vi "Insert Specifical Controls to [8,8] Array.vi"(7 "controls references":refnum<vi>[](array[refnum]), 8 "error in":errorcluster {"code" format="%.0x"}, 9 "2-D controls references":refnum<vi>[][](array[refnum]), 10 "indicators":refnum<vi>[](array[refnum]), 11 "controls":refnum<vi>[](array[refnum])) -> (0 "error out":errorcluster {"code" format="%.0x"}, 1 "2-D controls references out":refnum<vi>[][](array[refnum]), 2 "indicators out":refnum<vi>[](array[refnum]), 3 "controls out":refnum<vi>[](array[refnum]), 4 "controls references out":refnum<vi>[](array[refnum]))   [LabVIEW 2018, in "NISAST VI Scripting.lvlib" / "VI.lvlib" / "Front Panel.lvlib"]
uses:
  Front Panel.lvlib
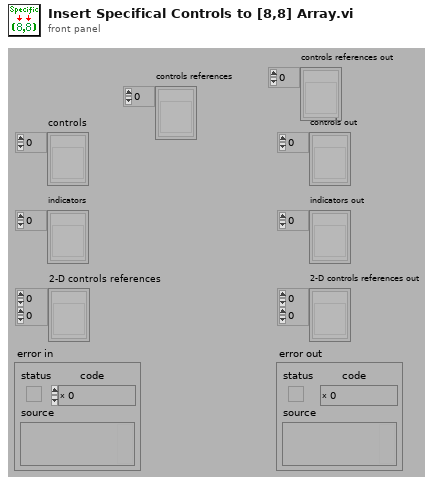
[diagram p1: front panel]
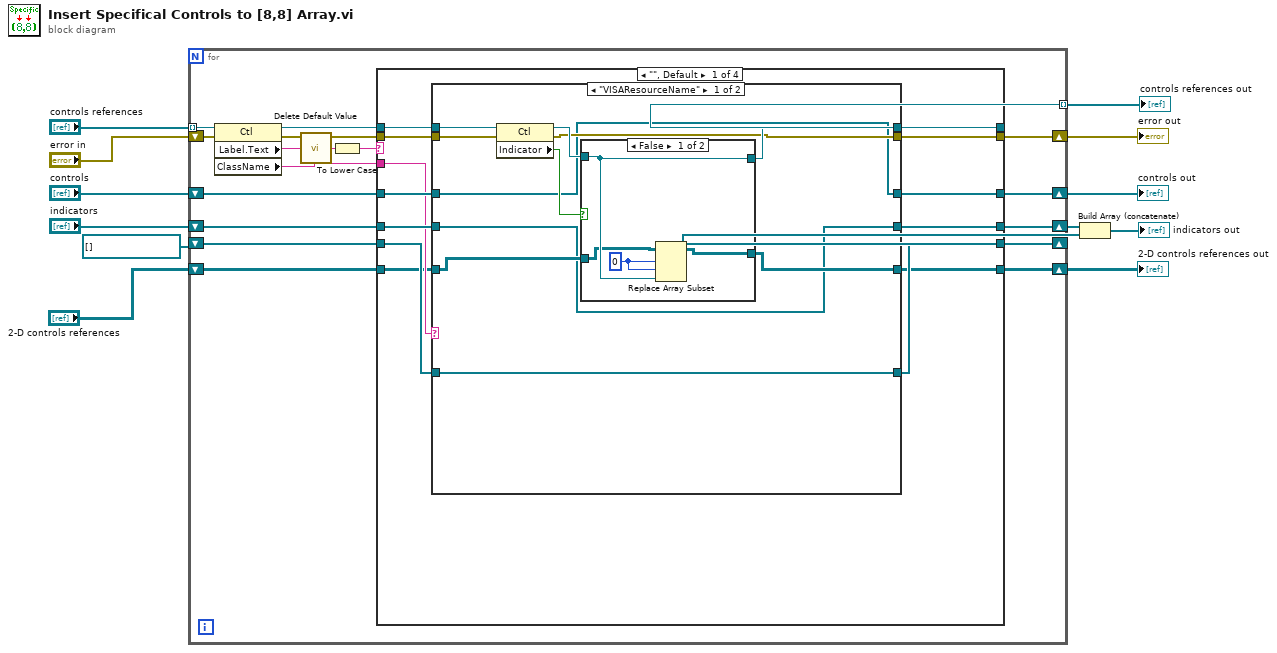
[diagram p0: block diagram]
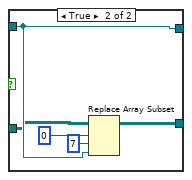
[diagram p2: hidden frame]
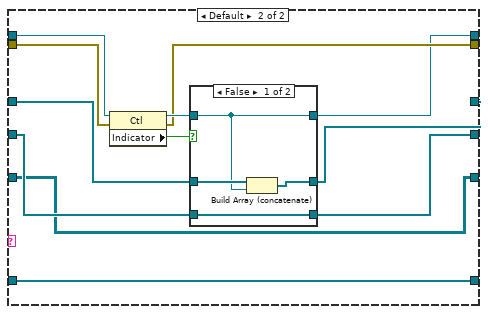
[diagram p3: hidden frame]
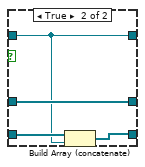
[diagram p4: hidden frame]
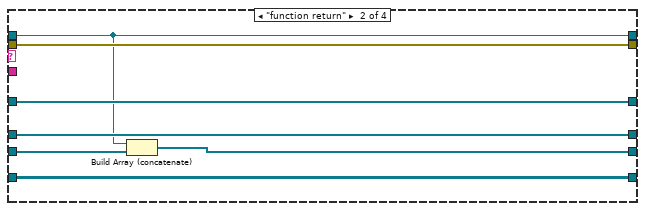
[diagram p5: hidden frame]
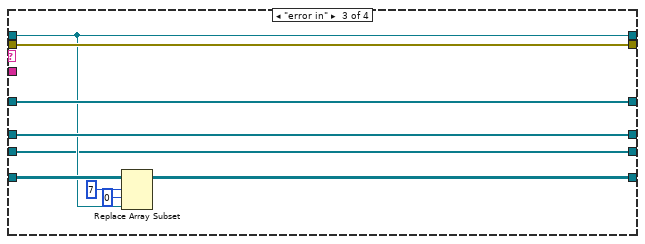
[diagram p6: hidden frame]
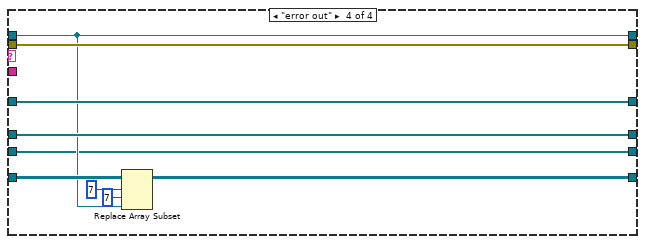
[diagram p7: hidden frame]
diagram:
  n1 = for {
    tunnel: "controls references" -> [w31] mode=indexing
    shift-right: [w28] -> w8
    shift-left: "2-D controls references" -> [w30]
    shift-right: [w27] -> w9
    shift-left: "controls" -> [w26]
    shift-right: [w24] -> w3
    shift-left: "indicators" -> [w25]
    shift-right: [w21] -> w6
    shift-left: "error in" -> [w22]
    tunnel: [w17] -> w5 mode=indexing
    shift-right: [w15] -> w1
    shift-left: refnum<vi>[] [] -> [w16]
    n2 = property class="Ctl"(reference=w31, error in=w22) -> (reference out=w29:refnum<vi>, error out=w23:errorcluster, "Label.Text"=w18:string, "ClassName"=w14:string)
    n3 = call "Delete Default Value.vi"("label or caption"=w18) -> ("naked label or caption"=w19:string)  [unwired: 4 out]
    n4 = To Lower Case(string=w19) -> (all lower case string=w20:string)
    n5 = case shown="\"\", Default" w20 {
      tunnel: w30 -> [w33 w91 w100 w109]
      tunnel: w29 -> [w44 w87 w93 w102]
      tunnel: [w32 w91 w97 w106] -> w28
      tunnel: [w43 w88 w96 w105] -> w27
      tunnel: w26 -> [w42 w88 w96 w105]
      tunnel: w25 -> [w41 w90 w95 w104]
      tunnel: [w40 w90 w95 w104] -> w24
      tunnel: w23 -> [w39 w89 w94 w103]
      tunnel: [w38 w89 w94 w103] -> w21
      tunnel: [w37 w87 w93 w102] -> w17
      tunnel: w16 -> [w35 w86 w92 w101]
      tunnel: [w34 w85 w92 w101] -> w15
      tunnel: w14 -> [w36 _ _ _]
      frame "", Default {
        n6 = case shown="\"VISAResourceName\"" w36 {
          tunnel: w44 -> [w50 w76]
          tunnel: [w46 w73] -> w43
          tunnel: w42 -> [w46 w72]
          tunnel: w41 -> [w45 w71]
          tunnel: [w45 w70] -> w40
          tunnel: w39 -> [w48 w69]
          tunnel: [w47 w68] -> w38
          tunnel: [w49 w67] -> w37
          tunnel: w35 -> [w53 w65]
          tunnel: [w53 w65] -> w34
          tunnel: w33 -> [w52 w66]
          tunnel: [w51 w66] -> w32
          frame "VISAResourceName" {
            n7 = property class="Ctl"(reference=w50, error in=w48) -> (reference out=w54:refnum<vi>, error out=w47:errorcluster, "Indicator"=w55:bool)
            n8 = case shown="False" w55 {
              tunnel: w54 -> [w57 w61]
              tunnel: [w59 w62] -> w51
              tunnel: [w57 w61] -> w49
              tunnel: w52 -> [w56 w60]
              frame False {
                w58 = 0 ("index (row)")
                n9 = Replace Array Subset(array=w56, new element=w57, index (row)=w58, index (col)=w58) -> (w59:refnum<vi>[][])
              }
              frame True {
                n10 = Replace Array Subset(array=w60, new element=w61, index (row)=0, index (col)=7 ("disabled index (col)")) -> (w62:refnum<vi>[][])
              }
            }
          }
          frame Default {
            n11 = property class="Ctl"(reference=w76, error in=w69) -> (reference out=w74:refnum<vi>, error out=w68:errorcluster, "Indicator"=w75:bool)
            n12 = case shown="False" w75 {
              tunnel: w74 -> [w77 w81]
              tunnel: [w80 w82] -> w73
              tunnel: w72 -> [w79 w82]
              tunnel: [w78 w84] -> w70
              tunnel: w71 -> [w78 w83]
              tunnel: [w77 w81] -> w67
              frame False {
                n13 = Build Array (concatenate)(w79, w77) -> (w80:refnum<vi>[])
              }
              frame True {
                n14 = Build Array (concatenate)(w83, w81) -> (w84:refnum<vi>[])
              }
            }
          }
        }
      }
      frame "function return" {
        n15 = Build Array (concatenate)(w87, w86) -> (w85:refnum<vi>[])
      }
      frame "error in" {
        n16 = Replace Array Subset(array=w100, new element=w93, index (row)=7 ("Disabled Index (row)"), index (col)=0 ("Disabled Index (col)")) -> (w97:refnum<vi>[][])
      }
      frame "error out" {
        n17 = Replace Array Subset(array=w109, new element=w102, index (row)=7 ("Disabled Index (row)"), index (col)=7 ("Disabled Index (col)")) -> (w106:refnum<vi>[][])
      }
    }
  }
  "controls out" <- w9
  "2-D controls references out" <- w8
  "error out" <- w6
  "controls references out" <- w5
  n18 = Build Array (concatenate)(w3, w1) -> (→"indicators out":refnum<vi>[])
